vi "GenericDCPowerSupply_Core.vi"(8 "error in":errorcluster, 10 "ctrl queue in":refnum<queue>) -> (0 "error out":errorcluster, 2 "ctrl queue out":refnum<queue>)   [LabVIEW 2014, in "GenericDCPowerSupply.lvlib"]
uses:
  <instrlib>/GenericDCPowerSupply/GenericDCPowerSupply.lvlib
  <instrlib>/GenericDCPowerSupply/Public/GenericDCPS-State.ctl
  <instrlib>/GenericDCPowerSupply/Public/Data/GenericDCPS-Configs.ctl
  <instrlib>/GenericDCPowerSupply/Public/Data/HVCh-Configs.ctl
  <vilib>/Utility/error.llb/Error Cluster From Error Code.vi
  <vilib>/ErrorRing/Error Ring.xnode
  <userlib>/Utility/ErrorLog_lib.lvlib
panel:
  out "Power Supply Monitoring":cluster{"Gauge":dbl, "Clamped":bool}[][](array[cluster]) {"Gauge" scale=-140.0..140.0 scale format="%#_6p"}
  in  "Configs":T1={"# Channels"=16, "VMax"=140, "VMin"=-140, "# Serial"=11, "PSHandle"=0, "IOPortNum"=0, "Enable"=FALSE, "ZeroShutdown"=TRUE, "Initialized"=TRUE, "Configs"=[{"MaxVolt"=140.0, "MinVolt"=-140.0, "SetPoint"=0.0, "Readout"=0.0, "Enable"=TRUE, "Channel"=0, "Clamped"=FALSE}, {"MaxVolt"=140.0, "MinVolt"=-140.0, "SetPoint"=0.0, "Readout"=0.0, "Enable"=TRUE, "Channel"=1, "Clamped"=FALSE}, {"MaxVolt"=140.0, "MinVolt"=-140.0, "SetPoint"=0.0, "Readout"=0.0, "Enable"=TRUE, "Channel"=2, "Clamped"=FALSE}, {"MaxVolt"=140.0, "MinVolt"=-140.0, "SetPoint"=0.0, "Readout"=0.0, "Enable"=TRUE, "Channel"=3, "Clamped"=FALSE}, {"MaxVolt"=140.0, "MinVolt"=-140.0, "SetPoint"=0.0, "Readout"=0.0, "Enable"=TRUE, "Channel"=4, "Clamped"=FALSE}, {"MaxVolt"=140.0, "MinVolt"=-140.0, "SetPoint"=0.0, "Readout"=0.0, "Enable"=TRUE, "Channel"=5, "Clamped"=FALSE}, {"MaxVolt"=140.0, "MinVolt"=-140.0, "SetPoint"=0.0, "Readout"=0.0, "Enable"=TRUE, "Channel"=6, "Clamped"=FALSE}, {"MaxVolt"=140.0, "MinVolt"=-140.0, "SetPoint"=0.0, "Readout"=0.0, "Enable"=TRUE, "Channel"=7, "Clamped"=FALSE}, {"MaxVolt"=140.0, "MinVolt"=-140.0, "SetPoint"=0.0, "Readout"=0.0, "Enable"=TRUE, "Channel"=8, "Clamped"=FALSE}, {"MaxVolt"=140.0, "MinVolt"=-140.0, "SetPoint"=0.0, "Readout"=0.0, "Enable"=TRUE, "Channel"=9, "Clamped"=FALSE}, {"MaxVolt"=140.0, "MinVolt"=-140.0, "SetPoint"=0.0, "Readout"=0.0, "Enable"=TRUE, "Channel"=10, "Clamped"=FALSE}, {"MaxVolt"=140.0, "MinVolt"=-140.0, "SetPoint"=0.0, "Readout"=0.0, "Enable"=TRUE, "Channel"=11, "Clamped"=FALSE}, {"MaxVolt"=140.0, "MinVolt"=-140.0, "SetPoint"=0.0, "Readout"=0.0, "Enable"=TRUE, "Channel"=12, "Clamped"=FALSE}, {"MaxVolt"=140.0, "MinVolt"=-140.0, "SetPoint"=0.0, "Readout"=0.0, "Enable"=TRUE, "Channel"=13, "Clamped"=FALSE}, {"MaxVolt"=140.0, "MinVolt"=-140.0, "SetPoint"=0.0, "Readout"=0.0, "Enable"=TRUE, "Channel"=14, "Clamped"=FALSE}, {"MaxVolt"=140.0, "MinVolt"=-140.0, "SetPoint"=0.0, "Readout"=0.0, "Enable"=TRUE, "Channel"=15, "Clamped"=FALSE}]}
  in  "Serial #":i32=11
  in  "VMax":i32=140
  in  "VMin":i32=-140
  in  "Quit":bool
  in  "SetAll":bool
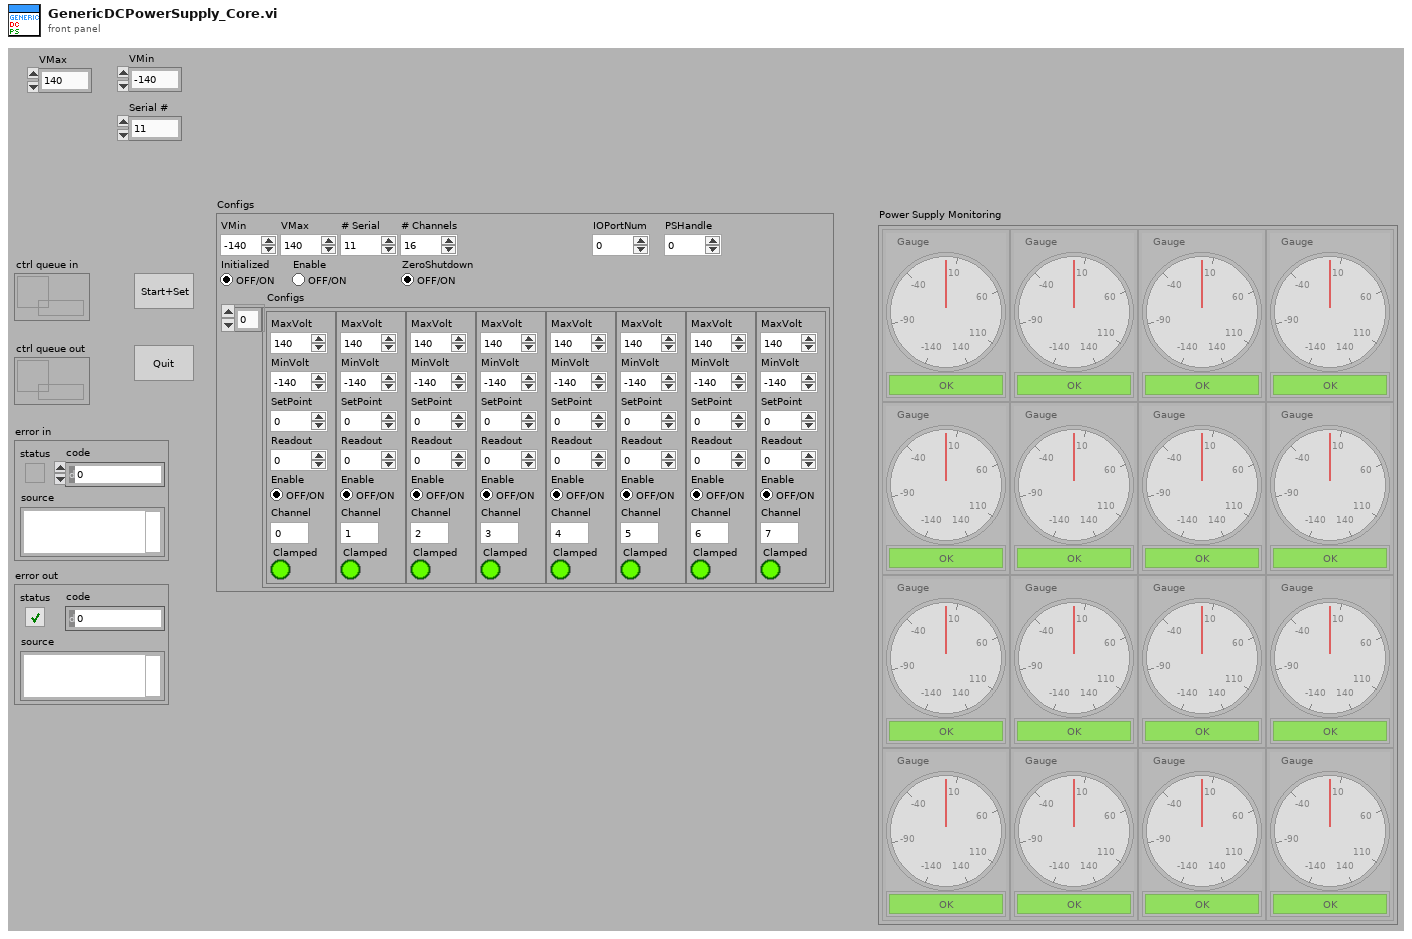
[diagram p1: front panel]
types:
  T1 = typedef "GenericDCPowerSupply.lvlib/GenericDCPS-Configs.ctl" = cluster{"# Channels":i32, "VMax":i32, "VMin":i32, "# Serial":i32, "PSHandle":i32, "IOPortNum":i32, "Enable":bool, "ZeroShutdown":bool, "Initialized":bool, "Configs":T2[]}
  T2 = typedef "GenericDCPowerSupply.lvlib/HVCh-Configs.ctl" = cluster{"MaxVolt":dbl, "MinVolt":dbl, "SetPoint":dbl, "Readout":dbl, "Enable":bool, "Channel":i32, "Clamped":bool}
  T3 = typedef "GenericDCPowerSupply.lvlib/GenericDCPS-State.ctl" = cluster{"State":enum16{"Enurmerate", "Open", "WriteVoltage", "ReadVoltage", "WriteAllChs", "ReadAllChs", "OnOff", "SetMinMax", "Close", "Quit", "=========", "GetStatus"}, "Para.":variant}
  T4 = enum16{"Enurmerate", "Open", "WriteVoltage", "ReadVoltage", "WriteAllChs", "ReadAllChs", "OnOff", "SetMinMax", "Close", "Quit", "=========", "GetStatus"}
  T5 = typedef "Ionwerks_HV_PowerSupply.lvlib/IWFS-Configs.ctl" = cluster{"# Channels":i32, "VMax":i32, "VMin":i32, "# Serial":i32, "PSHandle":i32, "IOPortNum":i32, "Enable":bool, "ZeroShutdown":bool, "Initialized":bool, "Configs":T6[]}
  T6 = typedef "Ionwerks_HV_PowerSupply.lvlib/HVCh-Configs.ctl" = cluster{"MaxVolt":dbl, "MinVolt":dbl, "SetPoint":dbl, "Readout":dbl, "Enable":bool, "Channel":i32, "Clamped":bool}
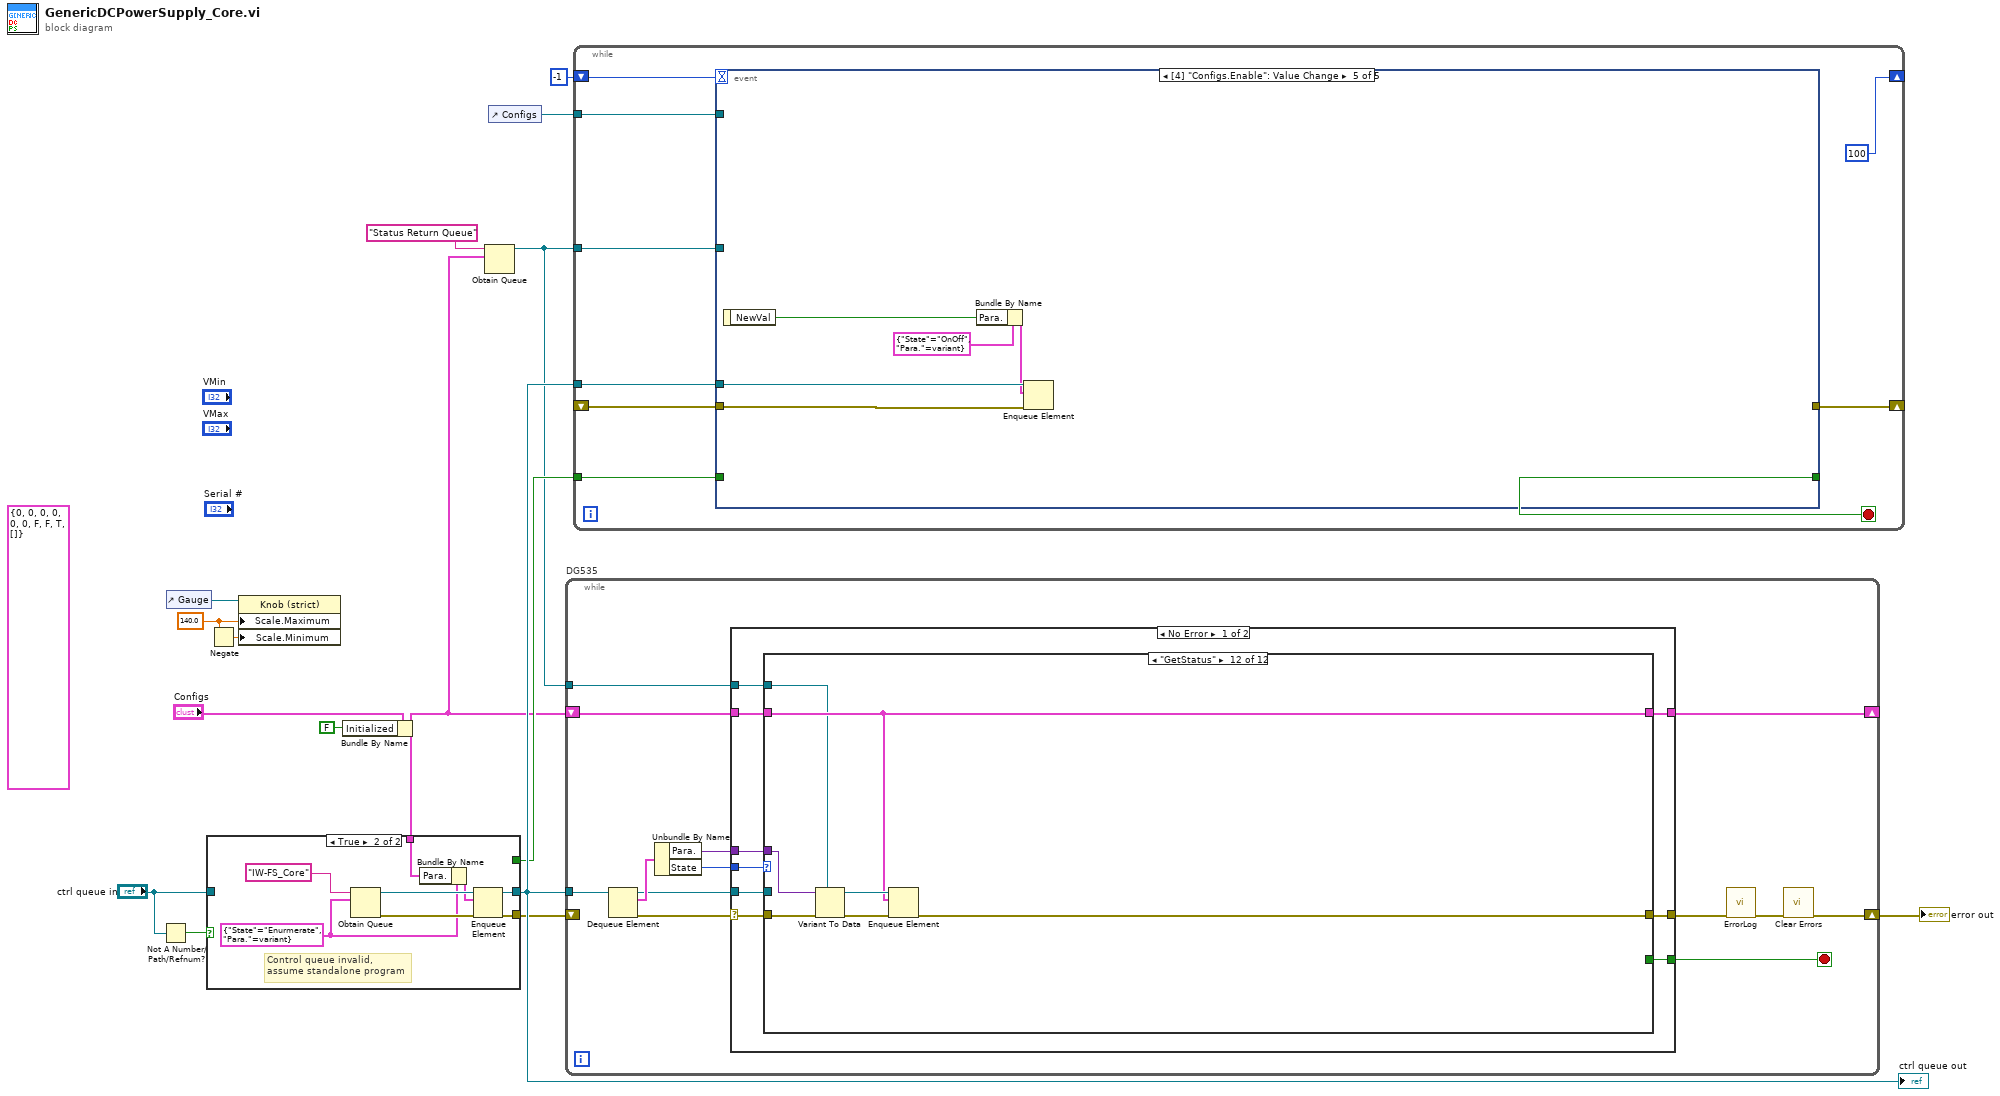
[diagram p0: block diagram]
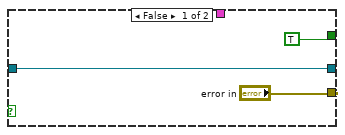
[diagram p2: hidden frame]
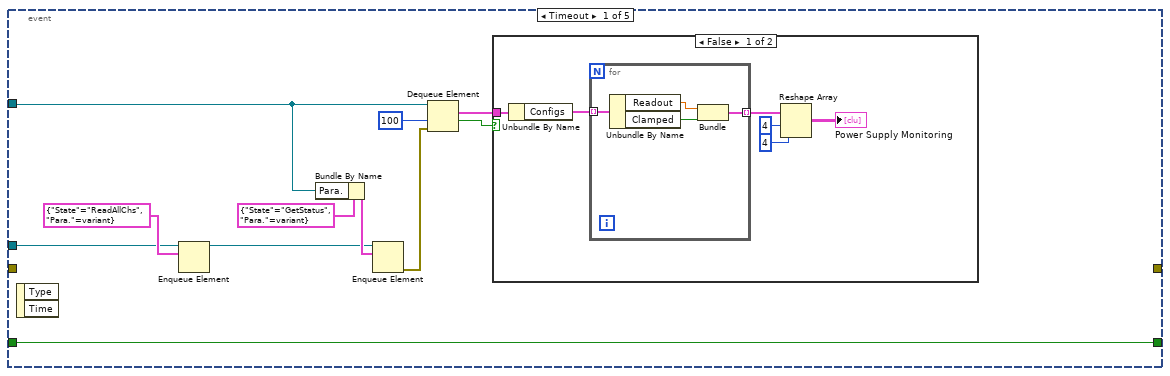
[diagram p3: hidden frame]
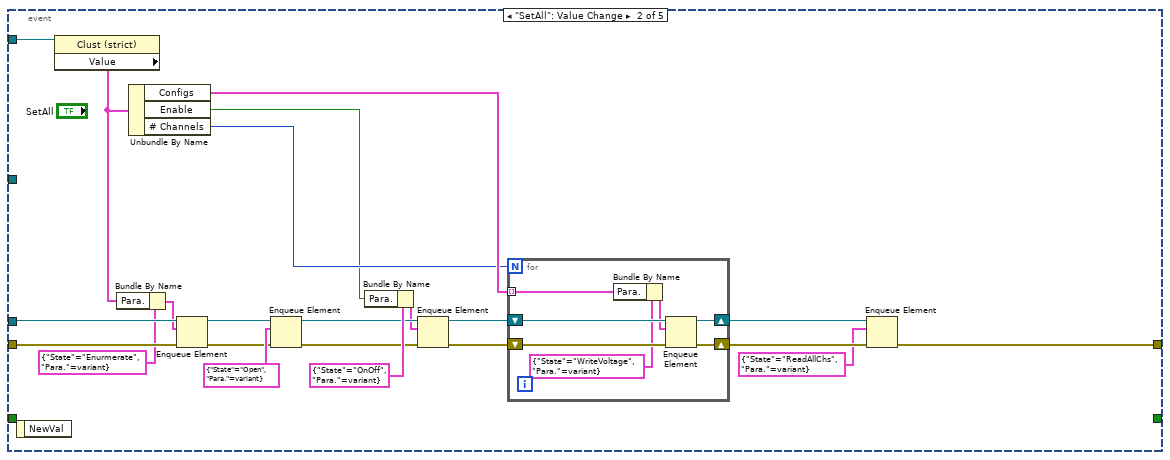
[diagram p5: hidden frame]
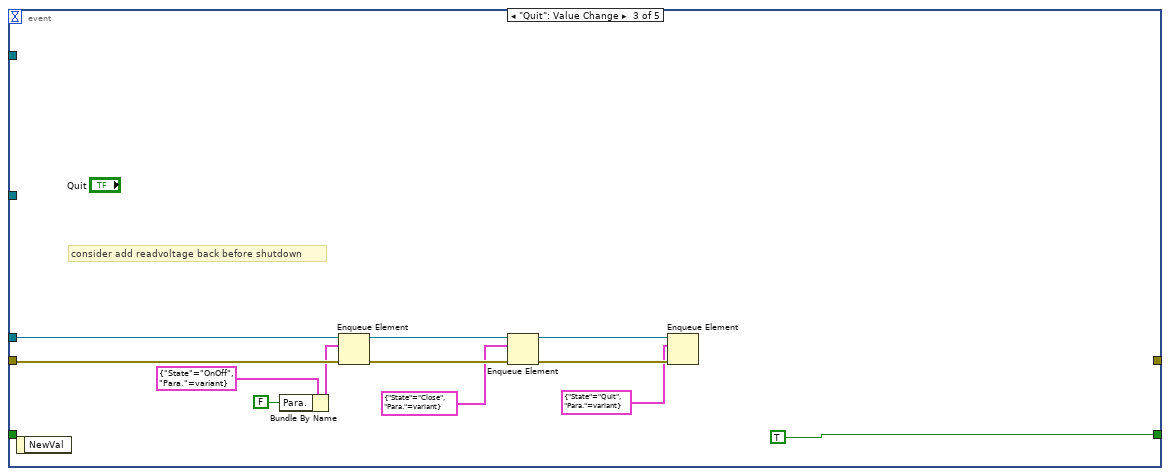
[diagram p6: hidden frame]
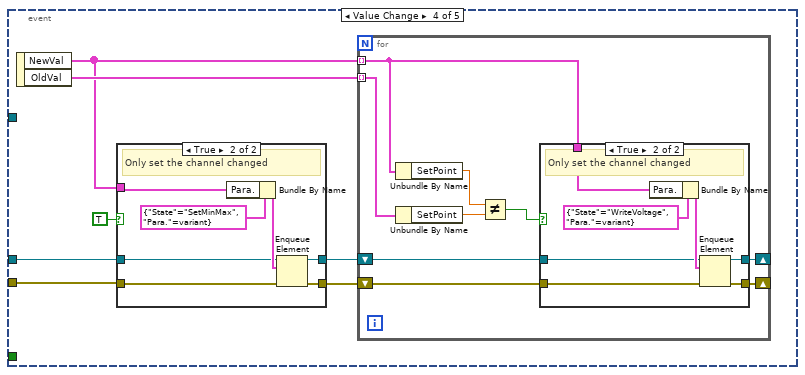
[diagram p7: hidden frame]
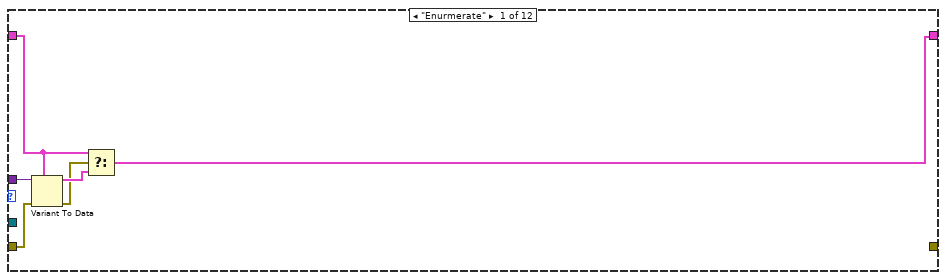
[diagram p10: hidden frame]
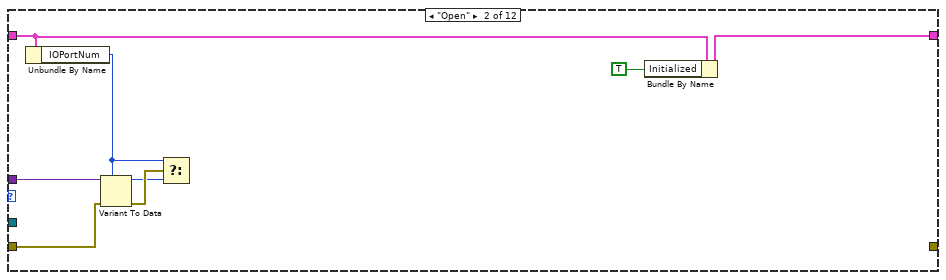
[diagram p11: hidden frame]
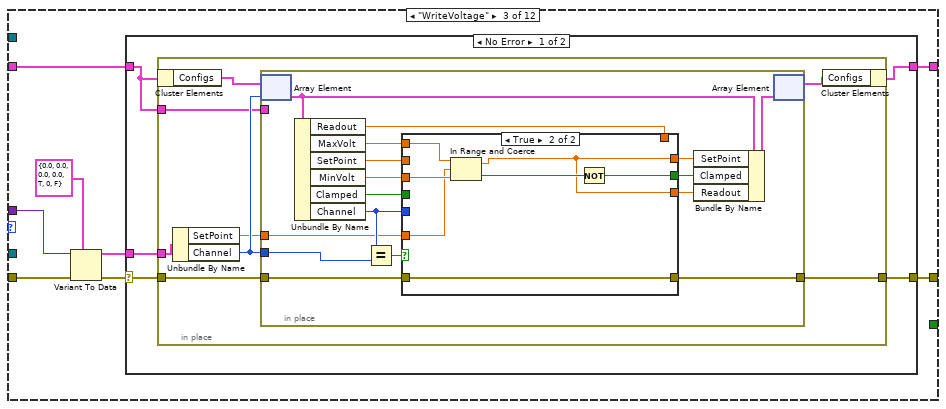
[diagram p12: hidden frame]
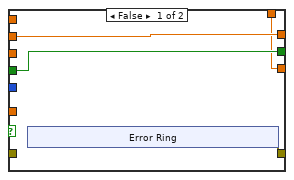
[diagram p13: hidden frame]
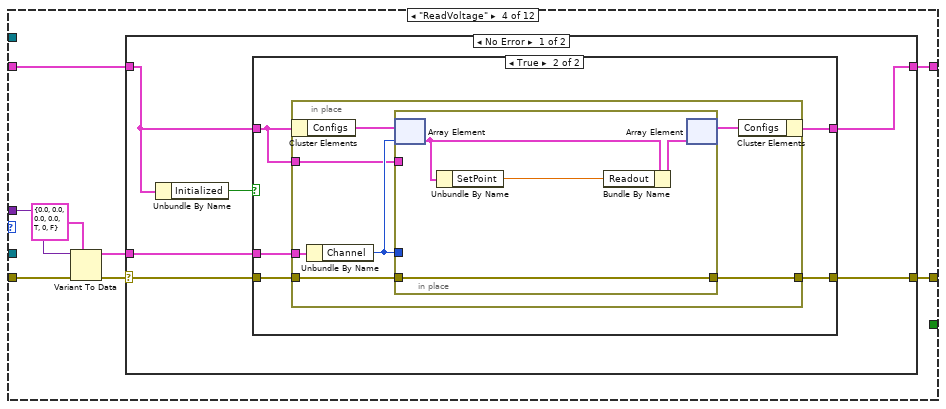
[diagram p15: hidden frame]
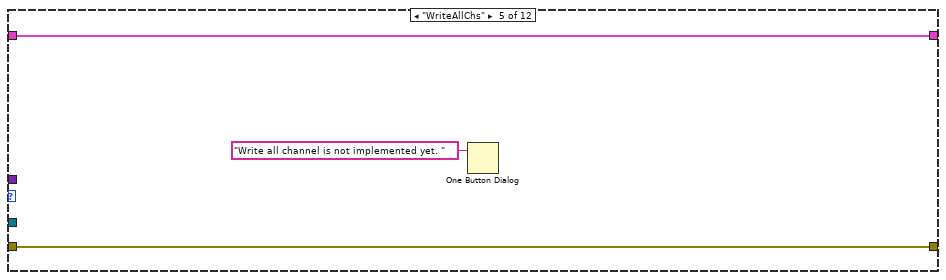
[diagram p18: hidden frame]
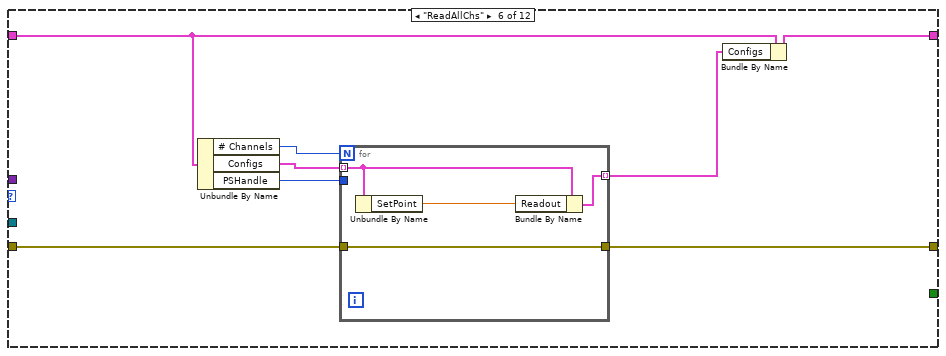
[diagram p19: hidden frame]
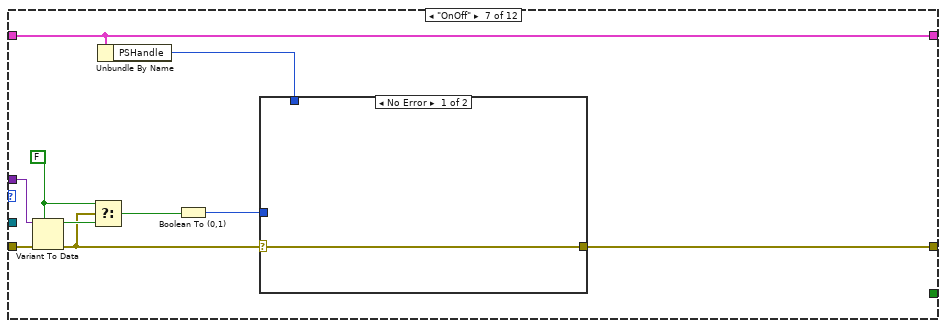
[diagram p20: hidden frame]
diagram:
  w6 = 140.0 ("Scale.Range:Maximum")
  (unwired) T1 {"# Channels"=0, "VMax"=0, "VMin"=0, "# Serial"=0, "PSHandle"=0, "IOPortNum"=0, "Enable"=FALSE, "ZeroShutdown"=FALSE, "Initialized"=TRUE, "Configs"=[]}
  n1 = Not A Number/Path/Refnum?(number/path/refnum="ctrl queue in") -> (NaN/Path/Refnum?=w15:bool)
  n2 = control-ref of="Gauge"() -> (w7:refnum<vi>)
  n3 = Negate(x=w6) -> (-x=w5:dbl)
  n4 = property class="Knob (strict)"(reference=w7, "Scale.Maximum"=w6, "Scale.Minimum"=w5) -> ()  [unwired: 1 in, 2 out]
  n5 = Bundle By Name(cluster="Configs", "Initialized"=FALSE) -> (w2:T1)
  n6 = case shown="True" w15 {
    tunnel: [w19 w24] -> w14
    tunnel: ["error in" w26] -> w13
    tunnel: "ctrl queue in" -> [w19 _]
    tunnel: w2 -> [_ w21]
    tunnel: [TRUE _] -> w12
    frame False {
    }
    frame True {
      w20 = T3 {"State"=enum."Enurmerate", "Para."=variant}
      # "Control queue invalid, \nassume standalone program"
      n7 = Obtain Queue(name (unnamed)="IW-FS_Core", element data type=w20) -> (queue out=w25:refnum<queue>, error out=w26:errorcluster)  [unwired: 3 in, 1 out]
      n8 = Bundle By Name(cluster=w20, "Para."=w21) -> (w22:T3)
      n9 = Enqueue Element(queue=w25, element=w22) -> (queue out=w24:refnum<queue>)  [unwired: 2 in, 2 out]
    }
  }
  "ctrl queue out" <- w14
  n10 = Obtain Queue(name (unnamed)="Status Return Queue", element data type=w2) -> (queue out=w3:refnum<queue>)  [unwired: 3 in, 2 out]
  n11 = control-ref of="Configs"() -> (w4:refnum<vi>)
  n12 = while "DG535" {
    tunnel: w14 -> [w39]
    shift-right: [w30] -> w16
    shift-left: w13 -> [_]
    shift-right: [w31] -> _
    shift-left: w2 -> [w32]
    tunnel: w3 -> [w27]
    stop <- w33 stop-if-true
    n13 = Dequeue Element(queue=w39) -> (queue out=w35:refnum<queue>, element=w38:T3, error out=w34:errorcluster)  [unwired: 2 in, 1 out]
    n14 = Unbundle By Name(w38) -> ("Para."=w36:variant, "State"=w37:T4)
    n15 = case shown="No Error" w34 {
      selector: w34 -> [w42 w269]
      tunnel: w37 -> [w48 _]
      tunnel: w36 -> [w47 _]
      tunnel: w35 -> [w46 _]
      tunnel: [w45 w269] -> w28
      tunnel: [w41 TRUE] -> w33
      tunnel: w32 -> [w44 w270]
      tunnel: [w43 w270] -> w31
      tunnel: w27 -> [w40 _]
      frame No Error {
        n16 = case shown="\"GetStatus\"" w48 {
          tunnel: w47 -> [w54 w62 w69 w124 _ _ w173 w188 _ _ _ w263]
          tunnel: w46 -> [_ _ _ _ _ _ _ _ _ _ _ _]
          tunnel: w42 -> [w53 w60 w68 w123 w154 w157 w172 w187 w234 w259 w261 w265]
          tunnel: [_ _ w63 w119 w154 w156 w168 w185 w233 w259 w261 w264] -> w45
          tunnel: w44 -> [w51 w59 w65 w118 w153 w162 w176 w182 w235 w258 w260 w267]
          tunnel: [w49 w61 w64 w120 w153 w159 w176 w181 w230 w258 w260 w267] -> w43
          tunnel: [_ _ _ _ _ _ _ _ _ TRUE _ _] -> w41
          tunnel: w40 -> [_ _ _ _ _ _ _ _ _ _ _ w262]
          frame "Enurmerate" {
            n17 = Variant To Data(error in=w53, type=w51, Variant=w54) -> (data=w52:T1, error out=w50:errorcluster)
            n18 = Select(t=w51, s=w50, f=w52) -> (s? t:f=w49:T1)
          }
          frame "Open" {
            n19 = Unbundle By Name(w59) -> ("IOPortNum"=w57:i32)
            n20 = Variant To Data(error in=w60, type=w57, Variant=w62) -> (data=w56:i32, error out=w58:errorcluster)
            n21 = Select(t=w57, s=w58, f=w56) -> ()  [unwired: 1 out]
            n22 = Bundle By Name(cluster=w59, "Initialized"=TRUE ("x < y?")) -> (w61:T1)
          }
          frame "WriteVoltage" {
            n23 = Variant To Data(error in=w68, type=T2 {"MaxVolt"=0.0, "MinVolt"=0.0, "SetPoint"=0.0, "Readout"=0.0, "Enable"=TRUE, "Channel"=0, "Clamped"=FALSE}, Variant=w69) -> (data=w66:T2, error out=w67:errorcluster)
            n24 = case shown="No Error" w67 {
              selector: w67 -> [w72 w117]
              tunnel: w66 -> [w74 _]
              tunnel: w65 -> [w71 w116]
              tunnel: [w75 w116] -> w64
              tunnel: [w73 w117] -> w63
              frame No Error {
                n25 = in-place {
                  in-place-border: w74 -> [w81]
                  in-place-border: [w79] -> w73
                  in-place-border: w72 -> [w78]
                  in-place-border: w71 -> [w77]
                  n26 = in-place-cluster #1(w71) -> ("Configs"=w83:T2[])
                  n27 = Unbundle By Name(w81) -> ("SetPoint"=w76:dbl, "Channel"=w80:i32)
                  n28 = in-place {
                    in-place-border: w80 -> [w99]
                    in-place-border: [w91] -> w79
                    in-place-border: w78 -> [w90]
                    in-place-border: w77 -> [_]
                    in-place-border: w76 -> [w86]
                    n29 = in-place-array #2(w83, w80) -> (w93:T2)
                    n30 = Unbundle By Name(w93) -> ("Readout"=w84:dbl, "MaxVolt"=w95:dbl, "SetPoint"=w97:dbl, "MinVolt"=w96:dbl, "Clamped"=w88:bool, "Channel"=w87:i32)
                    n31 = Equal?(x=w87, y=w99) -> (x = y?=w98:bool)
                    n32 = case shown="True" w98 {
                      tunnel: w97 -> [w103 _]
                      tunnel: w96 -> [_ w115]
                      tunnel: w95 -> [_ w114]
                      tunnel: [w103 w109] -> w92
                      tunnel: [w102 w112] -> w91
                      tunnel: w90 -> [_ w112]
                      tunnel: [w101 w111] -> w89
                      tunnel: w88 -> [w101 _]
                      tunnel: w87 -> [_ _]
                      tunnel: w86 -> [_ w110]
                      tunnel: [w100 w109] -> w85
                      tunnel: w84 -> [w100 _]
                      frame False {
                        n33 = xnode "Error Ring"() -> ("error out"=w102:errorcluster)
                      }
                      frame True {
                        n34 = In Range and Coerce(upper limit=w114, x=w110, lower limit=w115) -> (coerced(x)=w109:dbl, In Range?=w113:bool)
                        n35 = Not(x=w113) -> (.not. x?=w111:bool)
                      }
                    }
                    n36 = Bundle By Name(cluster=w93, "SetPoint"=w92, "Clamped"=w89, "Readout"=w85) -> (w94:T2)
                    n37 = in-place-array #2(w94) -> (w82:T2[])  [unwired: 1 out]
                  }
                  n38 = in-place-cluster #1("Configs"=w82) -> (w75:T1)
                }
              }
              frame Error {
              }
            }
          }
          frame "ReadVoltage" {
            n39 = Variant To Data(error in=w123, type=T2 {"MaxVolt"=0.0, "MinVolt"=0.0, "SetPoint"=0.0, "Readout"=0.0, "Enable"=TRUE, "Channel"=0, "Clamped"=FALSE}, Variant=w124) -> (data=w121:T2, error out=w122:errorcluster)
            n40 = case shown="No Error" w122 {
              selector: w122 -> [w128 w151]
              tunnel: w121 -> [w130 _]
              tunnel: w118 -> [w127 w150]
              tunnel: [w131 w150] -> w120
              tunnel: [w129 w151] -> w119
              frame No Error {
                n41 = Unbundle By Name(w127) -> ("Initialized"=w126:bool)
                n42 = case shown="True" w126 {
                  tunnel: [w133 w138] -> w131
                  tunnel: w130 -> [_ w137]
                  tunnel: [w132 w136] -> w129
                  tunnel: w128 -> [w132 w135]
                  tunnel: w127 -> [w133 w134]
                  frame False {
                  }
                  frame True {
                    n43 = in-place {
                      in-place-border: w137 -> [w143]
                      in-place-border: [w141] -> w136
                      in-place-border: w135 -> [w140]
                      in-place-border: w134 -> [w139]
                      n44 = in-place-cluster #3(w134) -> ("Configs"=w145:T2[])
                      n45 = Unbundle By Name(w143) -> ("Channel"=w142:i32)
                      n46 = in-place {
                        in-place-border: w142 -> [_]
                        in-place-border: [w148] -> w141
                        in-place-border: w140 -> [w148]
                        in-place-border: w139 -> [_]
                        n47 = in-place-array #4(w145, w142) -> (w147:T2)
                        n48 = Unbundle By Name(w147) -> ("SetPoint"=w146:dbl)
                        n49 = Bundle By Name(cluster=w147, "Readout"=w146) -> (w149:T2)
                        n50 = in-place-array #4(w149) -> (w144:T2[])  [unwired: 1 out]
                      }
                      n51 = in-place-cluster #3("Configs"=w144) -> (w138:T1)
                    }
                  }
                }
              }
              frame Error {
              }
            }
          }
          frame "WriteAllChs" {
            n52 = One Button Dialog(message="Write all channel is not implemented yet. ") -> ()  [unwired: 1 in, 1 out]
          }
          frame "ReadAllChs" {
            n53 = Unbundle By Name(w162) -> ("# Channels"=w155:i32, "Configs"=w160:T2[], "PSHandle"=w161:i32)
            n54 = for {
              N: w155 -> [_]
              tunnel: w157 -> [w166]
              tunnel: w161 -> [_]
              tunnel: [w166] -> w156
              tunnel: w160 -> [w164] mode=indexing
              tunnel: [w165] -> w158 mode=indexing
              n55 = Unbundle By Name(w164) -> ("SetPoint"=w163:dbl)
              n56 = Bundle By Name(cluster=w164, "Readout"=w163) -> (w165:T2)
            }
            n57 = Bundle By Name(cluster=w162, "Configs"=w158) -> (w159:T1)
          }
          frame "OnOff" {
            w174 = FALSE
            n58 = Variant To Data(error in=w172, type=w174, Variant=w173) -> (data=w175:bool, error out=w167:errorcluster)
            n59 = Select(t=w174, s=w167, f=w175) -> (s? t:f=w171:bool)
            n60 = Unbundle By Name(w176) -> ("PSHandle"=w169:i32)
            n61 = Boolean To (0,1)(Boolean=w171) -> (0, 1=w170:i16)
            n62 = case shown="No Error" w167 {
              selector: w167 -> [w177 w178]
              tunnel: w170 -> [_ _]
              tunnel: w169 -> [_ _]
              tunnel: [w177 w178] -> w168
              frame No Error {
              }
              frame Error {
              }
            }
          }
          frame "SetMinMax" {
            n63 = Unbundle By Name(w182) -> ("# Channels"=w183:i32, "Configs"=w179:T2[])
            n64 = Variant To Data(error in=w187, type=w179, Variant=w188) -> (data=w184:T2[], error out=w186:errorcluster)
            n65 = case shown="No Error" w186 {
              selector: w186 -> [w190 w223]
              tunnel: [w191 w223] -> w185
              tunnel: w184 -> [w194 _]
              tunnel: w183 -> [w193 _]
              tunnel: w179 -> [w192 w222]
              tunnel: [w189 w222] -> w180
              frame No Error {
                n66 = for {
                  N: w193 -> [_]
                  tunnel: w194 -> [w206] mode=indexing
                  tunnel: w192 -> [w200] mode=indexing
                  shift-right: [w202] -> w191
                  shift-left: w190 -> [w201]
                  tunnel: [w199] -> w189 mode=indexing
                  i -> [w204]
                  n67 = Unbundle By Name(w206) -> ("MaxVolt"=w197:dbl, "MinVolt"=w196:dbl, "Channel"=w205:i32)
                  n68 = Unbundle By Name(w200) -> ("MaxVolt"=w198:dbl, "MinVolt"=w195:dbl)
                  n69 = Equal?(x=w205, y=w204) -> (x = y?=w203:bool)
                  n70 = case shown="False" w203 {
                    tunnel: [w211 w221] -> w202
                    tunnel: w201 -> [_ w221]
                    tunnel: w200 -> [w209 w220]
                    tunnel: [w210 w219] -> w199
                    tunnel: w198 -> [w208 _]
                    tunnel: w197 -> [_ w218]
                    tunnel: w196 -> [_ w217]
                    tunnel: w195 -> [w207 _]
                    frame False {
                      n71 = xnode "Error Ring"() -> ("error out"=w211:errorcluster)
                      n72 = Bundle By Name(cluster=w209, "MaxVolt"=w208, "MinVolt"=w207) -> (w210:T2)
                    }
                    frame True {
                      n73 = Bundle By Name(cluster=w220, "MaxVolt"=w218, "MinVolt"=w217) -> (w219:T2)
                    }
                  }
                }
              }
              frame Error {
              }
            }
            n74 = Bundle By Name(cluster=w182, "Configs"=w180) -> (w181:T1)
          }
          frame "Close" {
            n75 = Unbundle By Name(w235) -> ("PSHandle"=w232:i32, "# Channels"=w231:i32, "Configs"=w228:T2[], "ZeroShutdown"=w226:bool, "Initialized"=w225:bool)
            n76 = case shown="True" w225 {
              tunnel: w234 -> [w236 w244]
              tunnel: [w236 w243] -> w233
              tunnel: w232 -> [_ w242]
              tunnel: w231 -> [_ w241]
              tunnel: w228 -> [w237 w240]
              tunnel: [w237 w239] -> w227
              tunnel: w226 -> [_ w238]
              frame False {
              }
              frame True {
                n77 = case shown="True" w238 {
                  tunnel: w244 -> [w245 w252]
                  tunnel: [w245 w251] -> w243
                  tunnel: w242 -> [_ w250]
                  tunnel: w241 -> [_ w249]
                  tunnel: w240 -> [w246 w248]
                  tunnel: [w246 w247] -> w239
                  frame False {
                  }
                  frame True {
                    # "Safety Feature: Shutdown all channel when closes."
                    n78 = for {
                      N: w249 -> [_]
                      tunnel: w252 -> [w256]
                      tunnel: w250 -> [_]
                      tunnel: [w256] -> w251
                      tunnel: w248 -> [w255] mode=indexing
                      tunnel: [w254] -> w247 mode=indexing
                      n79 = Bundle By Name(cluster=w255, "Readout"=0.0) -> (w254:T2)
                    }
                  }
                }
              }
            }
            n80 = Bundle By Name(cluster=w235, "PSHandle"=-1, "Configs"=w227, "Initialized"=FALSE) -> (w230:T1)
          }
          frame "Quit" {
          }
          frame "=========" {
          }
          frame "GetStatus" {
            n81 = Variant To Data(error in=w265, type=w262, Variant=w263) -> (data=w268:refnum<queue>, error out=w266:errorcluster)
            n82 = Enqueue Element(queue=w268, element=w267, error in (no error)=w266) -> (error out=w264:errorcluster)  [unwired: 1 in, 2 out]
          }
        }
      }
      frame Error {
      }
    }
    n83 = call <userlib>:"ErrorLog.vi"("error in (no error)"=w28) -> ("error out"=w29:errorcluster)  [unwired: 10 in]
    n84 = call <vilib>:"Clear Errors.vi"("error in (no error)"=w29) -> ("error out"=w30:errorcluster)  [unwired: 5 in, 1 out]
  }
  "error out" <- w16
  n85 = while {
    tunnel: w14 -> [w280]
    shift-right: [w279] -> _
    shift-left: _ -> [w278]
    tunnel: w12 -> [w276]
    shift-right: [100] -> _
    shift-left: -1 -> [w275]
    tunnel: w3 -> [w273]
    tunnel: w4 -> [w272]
    stop <- w277 stop-if-true
    n86 = event shown="[4] \"Configs.Enable\": Value Change" {
      selector: _ -> [_ _ _ _ _]
      dyn-events: _ -> [_ _ _ _ _]
      timeout: w275 -> [_ _ _ _ _]
      tunnel: w280 -> [w281 w323 w340 w349 w381]
      tunnel: [_ w319 _ _ _] -> w279
      tunnel: w278 -> [_ w322 w341 w344 w380]
      tunnel: [w291 _ TRUE _ _] -> w277
      tunnel: w276 -> [w291 _ _ _ _]
      tunnel: w273 -> [w288 _ _ _ _]
      tunnel: w272 -> [_ w318 _ _ _]
      event Timeout {
        n87 = event-data() -> ()  [unwired: 1 in, 2 out]
        n88 = Enqueue Element(queue=w281, element=T3 {"State"=enum."ReadAllChs", "Para."=variant}) -> (queue out=w282:refnum<queue>)  [unwired: 2 in, 2 out]
        n89 = Bundle By Name(cluster=T3 {"State"=enum."GetStatus", "Para."=variant} ("element"), "Para."=w288) -> (w289:T3)
        n90 = Enqueue Element(queue=w282, element=w289) -> (error out=w287:errorcluster)  [unwired: 2 in, 2 out]
        n91 = Dequeue Element(queue=w288, timeout in ms (-1)=100, error in (no error)=w287) -> (element=w286:T1, timed out?=w284:bool)  [unwired: 2 out]
        n92 = case shown="False" w284 {
          tunnel: w286 -> [w297 _]
          frame False {
            n93 = Unbundle By Name(w297) -> ("Configs"=w296:T2[])
            n94 = for {
              tunnel: w296 -> [w301] mode=indexing
              tunnel: [w298] -> w295 mode=indexing
              n95 = Unbundle By Name(w301) -> ("Readout"=w300:dbl, "Clamped"=w299:bool)
              n96 = Bundle("Readout"=w300, "Clamped"=w299) -> (w298:cluster{"Readout":dbl, "Clamped":bool})  [unwired: 1 in]
            }
            n97 = Reshape Array(w295, 4 ("dimension size"), 4 ("dimension size")) -> (→"Power Supply Monitoring":cluster{"Readout":dbl, "Clamped":bool}[][])
          }
          frame True {
          }
        }
      }
      event "SetAll": Value Change {
        n98 = event-data() -> ()  [unwired: 1 in, 1 out]
        n99 = property class="Clust (strict)"(reference=w318) -> ("Value"=w305:T5)  [unwired: 1 in, 2 out]
        n100 = Bundle By Name(cluster=T3 {"State"=enum."Enurmerate", "Para."=variant} ("element"), "Para."=w305) -> (w306:T3)
        n101 = Unbundle By Name(w305) -> ("Configs"=w317:T6[], "Enable"=w307:bool, "# Channels"=w316:i32)
        n102 = Enqueue Element(queue=w323, element=w306, error in (no error)=w322) -> (queue out=w313:refnum<queue>, error out=w312:errorcluster)  [unwired: 1 in, 1 out]
        n103 = Enqueue Element(queue=w313, element=T3 {"State"=enum."Open", "Para."=variant}, error in (no error)=w312) -> (queue out=w310:refnum<queue>, error out=w309:errorcluster)  [unwired: 1 in, 1 out]
        n104 = Bundle By Name(cluster=T3 {"State"=enum."OnOff", "Para."=variant} ("element"), "Para."=w307) -> (w308:T3)
        n105 = Enqueue Element(queue=w310, element=w308, error in (no error)=w309) -> (queue out=w303:refnum<queue>, error out=w304:errorcluster)  [unwired: 1 in, 1 out]
        n106 = for {
          N: w316 -> [_]
          shift-right: [w328] -> w320
          shift-left: w304 -> [w329]
          shift-right: [w327] -> w321
          shift-left: w303 -> [w330]
          tunnel: w317 -> [w324] mode=indexing
          n107 = Bundle By Name(cluster=T3 {"State"=enum."WriteVoltage", "Para."=variant} ("element"), "Para."=w324) -> (w326:T3)
          n108 = Enqueue Element(queue=w330, element=w326, error in (no error)=w329) -> (queue out=w327:refnum<queue>, error out=w328:errorcluster)  [unwired: 1 in, 1 out]
        }
        n109 = Enqueue Element(queue=w321, element=T3 {"State"=enum."ReadAllChs", "Para."=variant}, error in (no error)=w320) -> (error out=w319:errorcluster)  [unwired: 1 in, 2 out]
      }
      event "Quit": Value Change {
        # "consider add readvoltage back before shutdown"
        n110 = event-data() -> ()  [unwired: 1 in, 1 out]
        n111 = Bundle By Name(cluster=T3 {"State"=enum."OnOff", "Para."=variant}, "Para."=FALSE) -> (w334:T3)
        n112 = Enqueue Element(queue=w340, element=w334, error in (no error)=w341) -> (queue out=w337:refnum<queue>, error out=w336:errorcluster)  [unwired: 1 in, 1 out]
        n113 = Enqueue Element(queue=w337, element=T3 {"State"=enum."Close", "Para."=variant}, error in (no error)=w336) -> (queue out=w339:refnum<queue>, error out=w338:errorcluster)  [unwired: 1 in, 1 out]
        n114 = Enqueue Element(queue=w339, element=T3 {"State"=enum."Quit", "Para."=variant}, error in (no error)=w338) -> ()  [unwired: 1 in, 3 out]
      }
      event Value Change {
        n115 = event-data() -> ("NewVal"=w346:T2[], "OldVal"=w347:T2[])  [unwired: 1 in]
        n116 = case shown="True" TRUE {
          tunnel: w346 -> [_ w356]
          tunnel: w349 -> [w351 w355]
          tunnel: [w351 w354] -> w343
          tunnel: w344 -> [w350 w353]
          tunnel: [w350 w352] -> w348
          frame False {
          }
          frame True {
            # "Only set the channel changed"
            n117 = Bundle By Name(cluster=T3 {"State"=enum."SetMinMax", "Para."=variant} ("element"), "Para."=w356) -> (w358:T3)
            n118 = Enqueue Element(queue=w355, element=w358, error in (no error)=w353) -> (queue out=w354:refnum<queue>, error out=w352:errorcluster)  [unwired: 1 in, 1 out]
          }
        }
        n119 = for {
          tunnel: w346 -> [w364] mode=indexing
          tunnel: w347 -> [w367] mode=indexing
          shift-right: [w360] -> _
          shift-left: w348 -> [w361]
          shift-right: [w359] -> _
          shift-left: w343 -> [w362]
          n120 = Unbundle By Name(w364) -> ("SetPoint"=w366:dbl)
          n121 = Unbundle By Name(w367) -> ("SetPoint"=w365:dbl)
          n122 = Not Equal?(x=w366, y=w365) -> (x != y?=w363:bool)
          n123 = case shown="True" w363 {
            tunnel: w364 -> [_ w374]
            tunnel: w362 -> [w368 w373]
            tunnel: w361 -> [w369 w372]
            tunnel: [w369 w371] -> w360
            tunnel: [w368 w370] -> w359
            frame False {
            }
            frame True {
              # "Only set the channel changed"
              n124 = Bundle By Name(cluster=T3 {"State"=enum."WriteVoltage", "Para."=variant} ("element"), "Para."=w374) -> (w376:T3)
              n125 = Enqueue Element(queue=w373, element=w376, error in (no error)=w372) -> (queue out=w370:refnum<queue>, error out=w371:errorcluster)  [unwired: 1 in, 1 out]
            }
          }
        }
      }
      event Value Change {
        n126 = event-data() -> ("NewVal"=w379:bool)  [unwired: 1 in]
        n127 = Bundle By Name(cluster=T3 {"State"=enum."OnOff", "Para."=variant} ("element"), "Para."=w379) -> (w378:T3)
        n128 = Enqueue Element(queue=w381, element=w378, error in (no error)=w380) -> ()  [unwired: 1 in, 3 out]
      }
    }
  }
